vi "seleccion.vi"(8 "error in (no error)":errorcluster, 10 "Seleccion":string, 11 "UI Actor in":refnum<class "UI Actor.lvclass">) -> (0 "error out":errorcluster, 3 "UI Actor out":refnum<class "UI Actor.lvclass">)   [LabVIEW 2019, in "UI Actor.lvlib" / "UI Actor.lvclass"]
uses:
  UI Actor.lvclass
  UI Actor.lvclass/UI Actor.ctl
  Actor M Messages/Update M Msg/Update M Msg.lvclass/Update M Msg.ctl
  <vilib>/ActorFramework/Message Enqueuer/Message Enqueuer.lvclass/Message Enqueuer.ctl
  <vilib>/ActorFramework/Message Enqueuer/Enqueue.vi
  Actor M Messages/Update M Msg/Update M Msg.lvclass
  C:/Program Files (x86)/National Instruments/LabVIEW 2019/vi.lib/ActorFramework/Message/Message.lvclass
  <vilib>/ActorFramework/Message Priority Queue/Priority Enqueue.vi
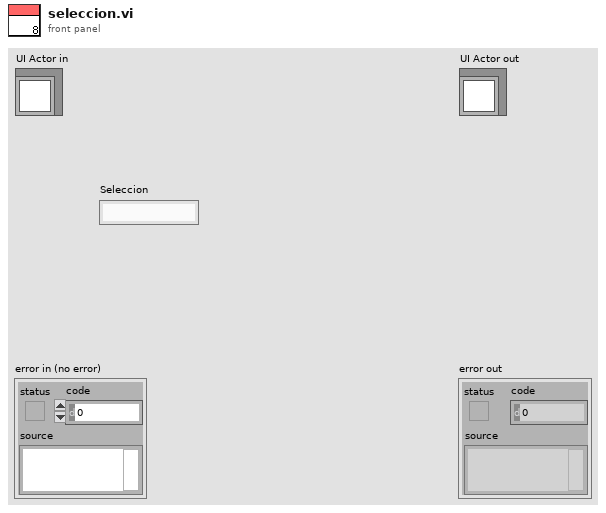
[diagram p1: front panel]
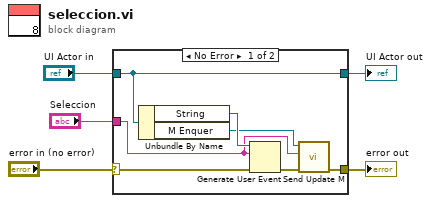
[diagram p0: block diagram]
diagram:
  n1 = case shown="No Error" "error in (no error)" {
    selector: "error in (no error)" -> [w10 w14]
    tunnel: [w6 w14] -> w4
    tunnel: [w12 w13] -> w2
    tunnel: "UI Actor in" -> [w12 w13]
    tunnel: "Seleccion" -> [w8 _]
    frame No Error {
      n2 = Unbundle By Name(w12) -> ("String"=w11:refnum<user-event>, "M Enquer"=w9:refnum<class "Message Enqueuer.lvclass">)
      n3 = Generate User Event(user event=w11, event data cluster=w8, error in=w10) -> (error out=w7:errorcluster)  [unwired: 1 in, 1 out]
      n4 = call "Send Update M.vi"("error in (no error)"=w7, "Update M"=w8, "Message Enqueuer"=w9) -> ("error out"=w6:errorcluster)  [unwired: 7 in, 1 out]
    }
    frame Error {
    }
  }
  "error out" <- w4
  "UI Actor out" <- w2
